vi "Rinocloud_HTTP_delete.vi"(8 "id":string) -> (0 "error out":errorcluster, 2 "body":string, 3 "headers":string)   [LabVIEW 2013]
uses:
  Rinocloud_global_variable.vi
  <vilib>/httpClient/POSTBuffer.vi
  <vilib>/httpClient/LabVIEWHTTPClient.lvlib
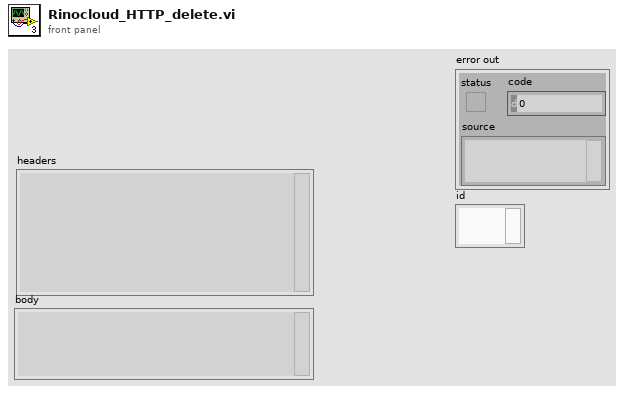
[diagram p1: front panel]
types:
  T1 = typedef "LabVIEWHTTPClient.lvlib/ClientHandle.ctl" = refnum<k1>
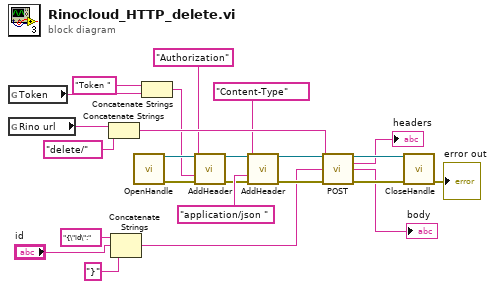
[diagram p0: block diagram]
diagram:
  n1 = global read "Rinocloud_global_variable.vi" "Token"() -> (w16:string)
  n2 = global read "Rinocloud_global_variable.vi" "Rino url"() -> (w22:string)
  n3 = Concatenate Strings(w22, "delete/" ("Combo Box 2")) -> (w24:string)
  n4 = Concatenate Strings("{\"id\":" ("string"), "id", "}" ("string")) -> (w1:string)
  n5 = call <vilib>:"OpenHandle.vi"() -> ("client handle out"=w20:T1, "error out"=w17:errorcluster)  [unwired: 14 in]
  n6 = Concatenate Strings("Token " ("value"), w16) -> (w18:string)
  n7 = call <vilib>:"AddHeader.vi"("client handle"=w20, "header"="Authorization" ("url"), "value"=w18, "error in (no error)"=w17) -> ("client handle out"=w9:T1, "error out"=w7:errorcluster)  [unwired: 10 in]
  n8 = call <vilib>:"AddHeader.vi"("client handle"=w9, "header"="Content-Type", "value"="application/json ", "error in (no error)"=w7) -> ("client handle out"=w8:T1, "error out"=w6:errorcluster)  [unwired: 10 in]
  n9 = call-poly <vilib>:"POST.vi"("client handle"=w8, "url"=w24, "buffer"=w1, "error in (no error)"=w6) -> ("client handle out"=w15:T1, "headers"=→"headers":string, "body"=→"body":string, "error out"=w14:errorcluster)  [unwired: 8 in]
  n10 = call <vilib>:"CloseHandle.vi"("client handle"=w15, "error in (no error)"=w14) -> ("error out"=→"error out":errorcluster)  [unwired: 13 in]
